vi "XY Graph Add Single Plot with Name.vi"(0 "XYGraph Ref in":T3, 1 "Scales (Default)":cluster{"X Scale":u32, "Y Scale":u32}, 2 "Plot Interpolation (Previous Plot's Style)":T2=7 items=["Point (.)", "Stepwise Right (--.)", "Line + Point (\\. /)", "Stepwise Left (.--)", "Stepwise Centered (-.-)", "Stepwise Vertical (|.|)", "Line (-)", "Use Previous Plot's Style"], 3 "Keep Existing Plots (T)":bool=TRUE, 5 "Plot":cluster{"X Array":dbl[], "Y Array":dbl[]}, 7 "Plot Metadata":variant, 9 "Plot Name (\"Plot\")":string, 11 "error in (no error)":errorcluster, 13 "Plot Color (Default)":u32(colorbox)=15781887, 14 "Point Style (Dot)":T1=enum."Dot") -> (4 "XY Graph Caption (or Label)":string, 8 "Plot Index":i32, 10 "Plot Name":string, 15 "error out":errorcluster)   [LabVIEW 2019]
uses:
  XY Graph Refnum.ctl
  LabVIEW Plot Interpolation.ctl
  Plot Point Style.ctl
  XY Graph Add-Ons.lvlib
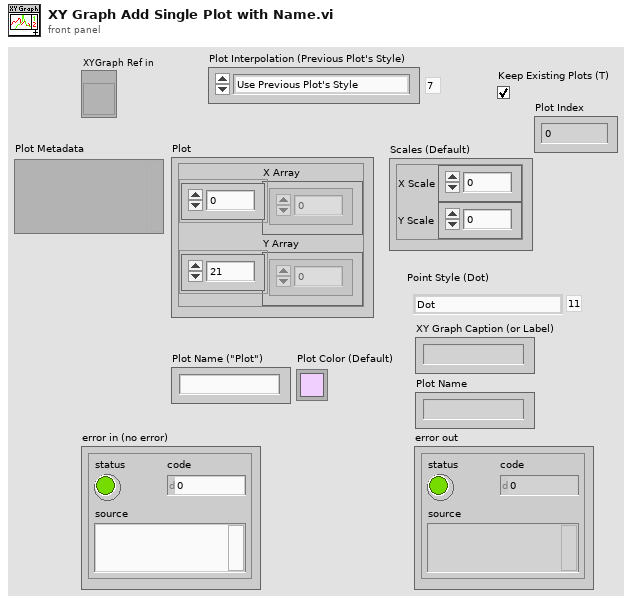
[diagram p1: front panel]
types:
  T1 = typedef "Plot Point Style.ctl" = enum16{"not defined", "None", "Empty Circle", "Filled Circle", "Thick Circle", "Dotted Circle", "Empty Square", "Filled Square", "Thick Square", "Dotted Square", "Small Filled Square", "Dot", "Cross", "Tiny Cross", "Large X", "Small x", "Diamond", "Small Empty Square"}
  T2 = typedef "LabVIEW Plot Interpolation.ctl" = u8
  T3 = typedef "XY Graph Add-Ons.lvlib/XY Graph Refnum.ctl" = refnum<vi>
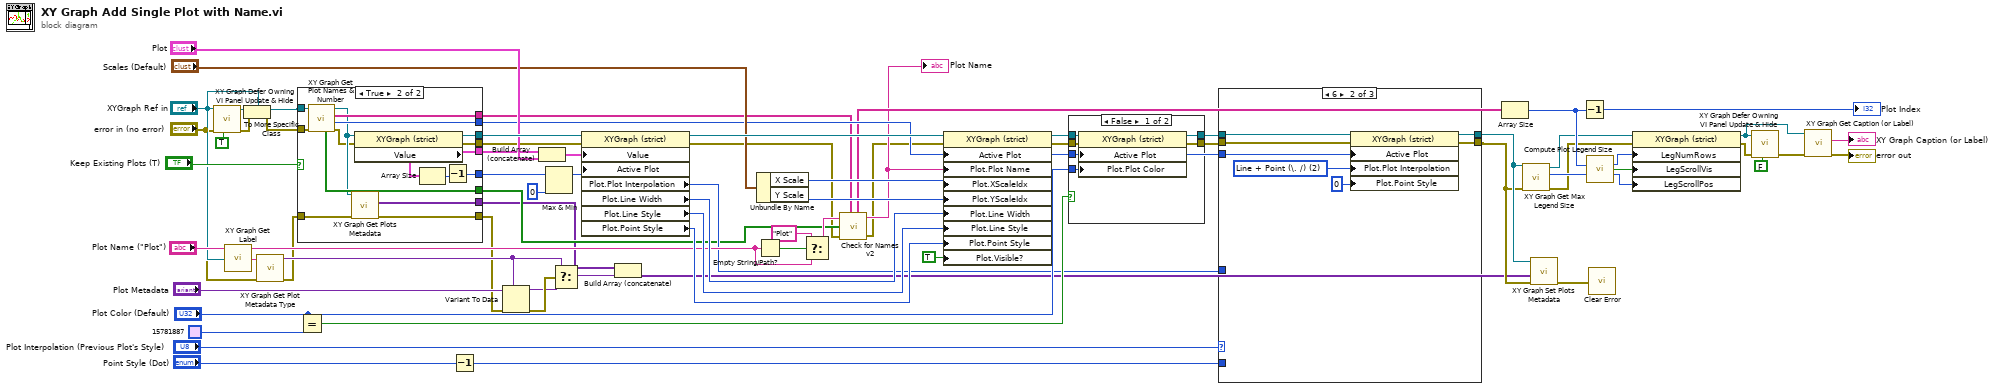
[diagram p0: block diagram]
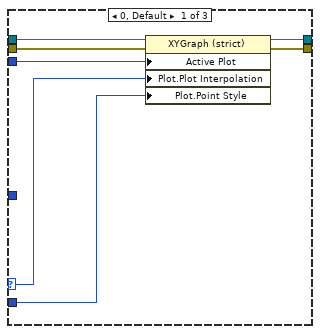
[diagram p3: hidden frame]
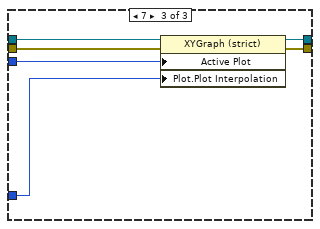
[diagram p4: hidden frame]
diagram:
  n1 = call "XY Graph Defer Owning VI Panel Update & Hide.vi"("Defer Owning Panel Update"=TRUE, "error in (no error)"="error in (no error)", "XY Graph Refnum in"="XYGraph Ref in") -> ("error out"=w29:errorcluster, "XY Graph Refnum out"=w36:refnum<vi>)  [unwired: 7 in]
  n2 = call "XY Graph Get Label.vi"("XYGraph"="XYGraph Ref in") -> ("Graph Label"=w10:string)  [unwired: 8 in]
  n3 = To More Specific Class(target class="XYGraph Ref in", reference=w36, error in=w29) -> (specific class reference=w30:T3, error out=w28:errorcluster)
  n4 = call "XY Graph Get Plot Metadata Type.vi"("Error In"="error in (no error)", "Graph Label"=w10) -> ("Error Out"=w2:errorcluster, "Plot Metadata Type"=w5:variant)  [unwired: 7 in, 1 out]
  n5 = case shown="True" "Keep Existing Plots (T)" {
    tunnel: w30 -> [w76 w91]
    tunnel: [w76 w90] -> w72
    tunnel: w28 -> [w75 w89]
    tunnel: [_ w88] -> w69
    tunnel: [_ w86] -> w68
    tunnel: [_ w85] -> w42
    tunnel: [_ w84] -> w51
    tunnel: [w75 w83] -> w46
    tunnel: [_ w82] -> w33
    tunnel: [_ w79] -> w13
    tunnel: w2 -> [w74 w78]
    tunnel: [w74 w77] -> w1
    frame False {
    }
    frame True {
      n6 = call "XY Graph Get Plot Names & Number.vi"("error in (no error)"=w89, "XYGraph in"=w91) -> ("error out"=w80:errorcluster, "# Plots"=w84:i32, "Plot Names"=w85:string[], "XYGraph out"=w81:T3, "Empty Plots?"=w82:bool[])  [unwired: 5 in]
      n7 = call "XY Graph Get Plots Metadata.vi"("Error In"=w78, "XYGraph Refnum"=w81) -> ("Error Out"=w77:errorcluster, "Plots Metadata"=w79:variant[])  [unwired: 6 in, 2 out]
      n8 = property class="XYGraph (strict)"(reference=w81, error in=w80) -> (reference out=w90:T3, error out=w83:errorcluster, "Value"=w88:cluster{"X Array":dbl[], "Y Array":dbl[]}[])
      n9 = Array Size(array=w88) -> (size(s)=w87:i32)
      n10 = Decrement(x=w87) -> (x-1=w86:i32)
    }
  }
  n11 = Equal?(x="Plot Color (Default)", y=u32 15781887 ("Plot Color (Default)")) -> (x = y?=w55:bool)
  n12 = Decrement(x="Point Style (Dot)") -> (x-1=w38:T1)
  n13 = Variant To Data(error in=w1, type=w5, Variant="Plot Metadata") -> (data=w4:variant, error out=w6:errorcluster)
  n14 = Build Array (concatenate)(w69, "Plot") -> (w73:cluster{"X Array":dbl[], "Y Array":dbl[]}[])
  n15 = Max & Min(x=w68, y=0) -> (max(x,y)=w48:i32)  [unwired: 1 out]
  n16 = Select(t=w5, s=w6, f=w4) -> (s? t:f=w3:variant)
  n17 = property class="XYGraph (strict)"(reference=w72, error in=w46, "Value"=w73, "Active Plot"=w48) -> (reference out=w71:T3, error out=w32:errorcluster, "Plot.Plot Interpolation"=w49:u8, "Plot.Line Width"=w67:u8, "Plot.Line Style"=w66:u8, "Plot.Point Style"=w65:u8)
  n18 = Build Array (concatenate)(w13, w3) -> (w12:variant[])
  n19 = Unbundle By Name("Scales (Default)") -> ("X Scale"=w64:u32, "Y Scale"=w63:u32)
  n20 = Empty String/Path?(string/path="Plot Name (\"Plot\")") -> (empty?=w62:bool)
  n21 = Select(t="Plot", s=w62, f="Plot Name (\"Plot\")") -> (s? t:f=w40:string)
  n22 = call "Check for Names v2.vi"("New Name"=w40, "Name List"=w42, "Empty Plots?"=w33, "Error In"=w32) -> ("New Name List"=w41:string[], "New Name"=w39:string, "Error Out"=w31:errorcluster)  [unwired: 2 in, 1 out]
  "Plot Name" <- w39
  n23 = property class="XYGraph (strict)"(reference=w71, error in=w31, "Active Plot"=w51, "Plot.Plot Name"=w39, "Plot.XScaleIdx"=w64, "Plot.YScaleIdx"=w63, "Plot.Line Width"=w67, "Plot.Line Style"=w66, "Plot.Point Style"=w65, "Plot.Visible?"=TRUE ("Plot.Visible")) -> (reference out=w57:T3, error out=w56:errorcluster)
  n24 = case shown="False" w55 {
    tunnel: w57 -> [w97 w99]
    tunnel: [w96 w99] -> w53
    tunnel: w56 -> [w95 w98]
    tunnel: [w94 w98] -> w52
    tunnel: w51 -> [w93 _]
    tunnel: "Plot Color (Default)" -> [w92 _]
    frame False {
      n25 = property class="XYGraph (strict)"(reference=w97, error in=w95, "Active Plot"=w93, "Plot.Plot Color"=w92) -> (reference out=w96:T3, error out=w94:errorcluster)
    }
    frame True {
    }
  }
  n26 = case shown="6" "Plot Interpolation (Previous Plot's Style)" {
    selector: "Plot Interpolation (Previous Plot's Style)" -> [w101 _ _]
    tunnel: w53 -> [w106 w113 w119]
    tunnel: [w105 w112 w118] -> w15
    tunnel: w52 -> [w104 w111 w117]
    tunnel: [w103 w110 w116] -> w14
    tunnel: w51 -> [w102 w109 w115]
    tunnel: w49 -> [_ _ w114]
    tunnel: w38 -> [w100 _ _]
    frame 0, Default {
      n27 = property class="XYGraph (strict)"(reference=w106, error in=w104, "Active Plot"=w102, "Plot.Plot Interpolation"=w101, "Plot.Point Style"=w100) -> (reference out=w105:T3, error out=w103:errorcluster)
    }
    frame 6 {
      w108 = T2 2 items=["Point (.)", "Stepwise Right (--.)", "Line + Point (\\. /)", "Stepwise Left (.--)", "Stepwise Centered (-.-)", "Stepwise Vertical (|.|)", "Line (-)", "Use Previous Plot's Style"] ("Plot Interpolation (Previous Plot's Style)")
      n28 = property class="XYGraph (strict)"(reference=w113, error in=w111, "Active Plot"=w109, "Plot.Plot Interpolation"=w108, "Plot.Point Style"=u8 0) -> (reference out=w112:T3, error out=w110:errorcluster)
    }
    frame 7 {
      n29 = property class="XYGraph (strict)"(reference=w119, error in=w117, "Active Plot"=w115, "Plot.Plot Interpolation"=w114) -> (reference out=w118:T3, error out=w116:errorcluster)
    }
  }
  n30 = Array Size(array=w41) -> (size(s)=w26:i32)
  n31 = call "XY Graph Get Max Legend Size.vi"("Error In"=w14, "XYGraph Refnum"=w15) -> ("Error Out"=w20:errorcluster, "Max Legend Size"=w27:i32, "XYGraph Refnum"=w21:T3)  [unwired: 6 in, 1 out]
  n32 = call "XY Graph Set Plots Metadata.vi"("error in (no error)"=w14, "Plots Metadata"=w12, "XY Graph Refnum"=w15) -> ("error out"=w11:errorcluster)  [unwired: 7 in, 1 out]
  n33 = Decrement(x=w26) -> (x-1=→"Plot Index":i32)
  n34 = call "Compute Plot Legend Size.vi"("# Plots"=w26, "Max Legend Size"=w27) -> ("LegNumRows"=w25:u32, "LegScrollVis"=w24:bool, "LegScrollPos"=w23:u32)  [unwired: 11 in]
  n35 = call "Clear Error.vi"("Error In"=w11) -> ()  [unwired: 8 in, 1 out]
  n36 = property class="XYGraph (strict)"(reference=w21, error in=w20, "LegNumRows"=w25, "LegScrollVis"=w24, "LegScrollPos"=w23) -> (reference out=w17:T3, error out=w34:errorcluster)
  n37 = call "XY Graph Defer Owning VI Panel Update & Hide.vi"("Defer Owning Panel Update"=FALSE, "error in (no error)"=w34, "XY Graph Refnum in"=w17) -> ("error out"=w18:errorcluster)  [unwired: 7 in, 1 out]
  n38 = call "XY Graph Get Caption (or Label).vi"("error in (no error)"=w18, "XYGraph in"=w17) -> ("error out"=→"error out":errorcluster, "Caption (or Label) Text"=→"XY Graph Caption (or Label)":string)  [unwired: 7 in, 1 out]
